vi "CLSUIP_ShiftTerminalBounds.vi"(1 "Terminal Bounds":T1(array[cluster]), 2 "Indices":i32[](array[numeric]), 3 "Shift Amount":i32) -> (0 "Terminal Bounds out":T1(array[cluster]))   [LabVIEW 2021, in "MemberVICreation.lvlib" / "VIRetooler.lvclass"]
uses:
  <resource>/Framework/Providers/LVClassLibrary/NewAccessors/VIRetooler/VIRetooler.lvclass
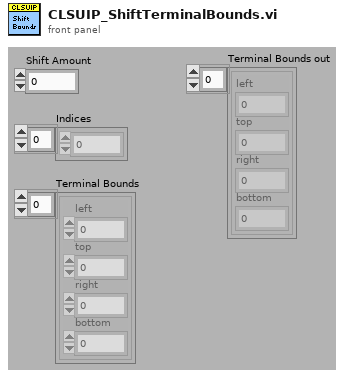
[diagram p1: front panel]
types:
  T1 = cluster{"left":i16, "top":i16, "right":i16, "bottom":i16}[]
  T2 = cluster{"left":i16, "top":i16, "right":i16, "bottom":i16}
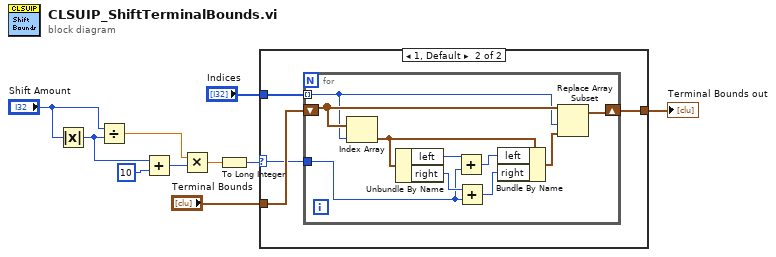
[diagram p0: block diagram]
diagram:
  n1 = Absolute Value(x="Shift Amount") -> (abs(x)=w5:i32)
  n2 = Divide(x="Shift Amount", y=w5) -> (x/y=w2:dbl)
  n3 = Add(x=w5, y=10) -> (x+y=w3:i32)
  n4 = Multiply(x=w2, y=w3) -> (x*y=w4:dbl)
  n5 = To Long Integer(number=w4) -> (32bit integer=w1:i32)
  n6 = case shown="1, Default" w1 {
    selector: w1 -> [_ w12]
    tunnel: [w11 w15] -> w10
    tunnel: "Indices" -> [_ w14]
    tunnel: "Terminal Bounds" -> [w11 w13]
    frame 0 {
    }
    frame 1, Default {
      n7 = for {
        tunnel: w14 -> [w24] mode=indexing
        shift-right: [w16] -> w15
        shift-left: w13 -> [w25]
        tunnel: w12 -> [w17]
        n8 = Index Array(array=w25, index=w24) -> (element=w22:T2)
        n9 = Unbundle By Name(w22) -> ("left"=w21:i16, "right"=w20:i16)
        n10 = Add(x=w21, y=w17) -> (x+y=w19:i32)
        n11 = Add(x=w20, y=w17) -> (x+y=w18:i32)
        n12 = Bundle By Name(cluster=w22, "left"=w19, "right"=w18) -> (w23:T2)
        n13 = Replace Array Subset(array=w25, new element=w23, index=w24) -> (w16:T1)
      }
    }
  }
  "Terminal Bounds out" <- w10
